vi "Wavefrom Subset from Cursors.vi"(8 "Error In":errorcluster, 9 "Waveform In":waveform(dbl), 11 "Waveform Graph":refnum<vi>) -> (0 "Error Out":errorcluster, 1 "Waveform Subsets":waveform(dbl)[](array[waveform]))   [LabVIEW 2017]
uses:
  <vilib>/Waveform/WDTOps.llb/WDT Waveform Duration DBL.vi
  <vilib>/Waveform/WDTOps.llb/WDT Get Waveform Subset DBL.vi
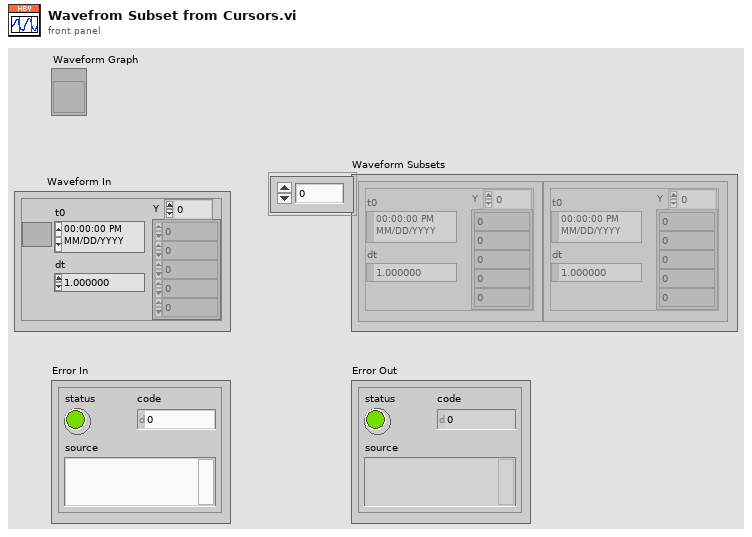
[diagram p1: front panel]
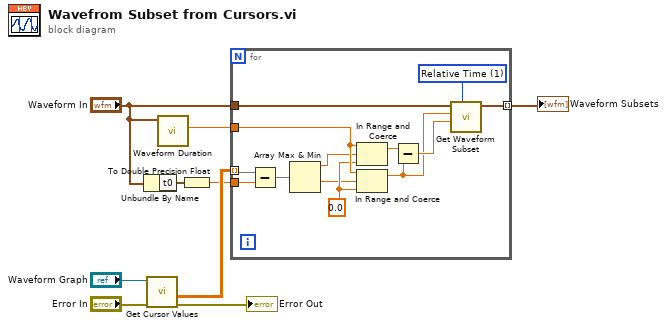
[diagram p0: block diagram]
diagram:
  n1 = Unbundle By Name("Waveform In") -> ("t0"=w6:timestamp)
  n2 = call "Get Cursor Values.vi"("error in (no error)"="Error In", "Waveform Graph Ref"="Waveform Graph") -> ("error out"=→"Error Out":errorcluster, "Cursor values"=w8:dbl[][])  [unwired: 7 in]
  n3 = call-poly <vilib>:"Waveform Duration.vi"("waveform in"="Waveform In") -> ("duration"=w9:dbl)  [unwired: 8 in, 2 out]
  n4 = To Double Precision Float(number=w6) -> (double precision float=w7:dbl)
  n5 = for {
    tunnel: w9 -> [w19]
    tunnel: w8 -> [w14] mode=indexing
    tunnel: w7 -> [w13]
    tunnel: "Waveform In" -> [w11]
    tunnel: [w10] -> w2 mode=indexing
    w17 = 0.0 ("lower limit")
    w12 = u16 1 items=["Samples", "Relative Time"] ("start/duration format")
    n6 = Subtract(x=w14, y=w13) -> (x-y=w15:dbl[])
    n7 = Array Max & Min(array=w15) -> (max value=w18:dbl, min value=w16:dbl)  [unwired: 2 out]
    n8 = In Range and Coerce(upper limit=w19, x=w18, lower limit=w17) -> (coerced(x)=w20:dbl)  [unwired: 1 out]
    n9 = In Range and Coerce(upper limit=w19, x=w16, lower limit=w17) -> (coerced(x)=w21:dbl)  [unwired: 1 out]
    n10 = Subtract(x=w20, y=w21) -> (x-y=w22:dbl)
    n11 = call-poly <vilib>:"Get Waveform Subset.vi"("start/duration format"=w12, "duration"=w22, "start samples/time"=w21, "waveform in"=w11) -> ("waveform out"=w10:waveform(dbl))  [unwired: 2 in, 3 out]
  }
  "Waveform Subsets" <- w2
